vi "average_line.vi"(9 "data-pts-per-line":i32, 10 "raw-data-row":dbl[](array[numeric]), 11 "number-of-pixels":i32) -> (3 "avg-data-row":dbl[](array[numeric]))   [LabVIEW 2015]
uses:
  <vilib>/Analysis/baseanly.llb/Mean (DBL).vi
  <vilib>/Analysis/NI_AALBase.lvlib
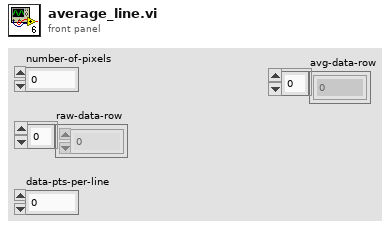
[diagram p1: front panel]
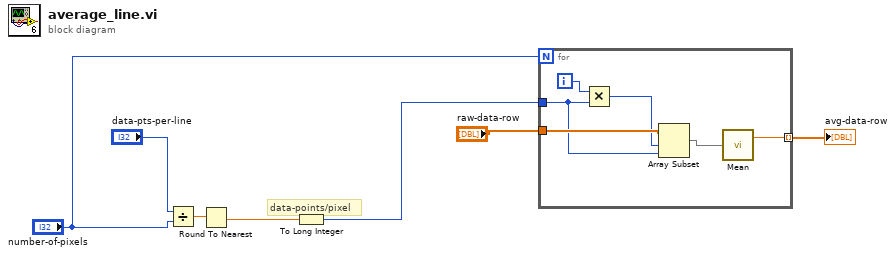
[diagram p0: block diagram]
diagram:
  # "data-points/pixel"
  n1 = Divide(x="data-pts-per-line", y="number-of-pixels") -> (x/y=w5:dbl)
  n2 = Round To Nearest(number=w5) -> (nearest integer value=w4:dbl)
  n3 = To Long Integer(number=w4) -> (32bit integer=w2:i32)
  n4 = for {
    N: "number-of-pixels" -> [_]
    tunnel: "raw-data-row" -> [w12]
    tunnel: [w10] -> w7 mode=indexing
    tunnel: w2 -> [w9]
    i -> [w13]
    n5 = Multiply(x=w13, y=w9) -> (x*y=w11:i32)
    n6 = Array Subset(array=w12, index=w11, length=w9) -> (w8:dbl[])
    n7 = call-poly <vilib>:"Mean.vi"("X"=w8) -> ("mean"=w10:dbl)  [unwired: 1 out]
  }
  "avg-data-row" <- w7
